vi "SR400_setting.vi"(4 "Counter B Input":enum16{"10 MHz", "INPUT 1", "INPUT 2", "TRIG"}(ring)=enum."INPUT 1", 5 "Counter A Input":enum16{"10 MHz", "INPUT 1", "INPUT 2", "TRIG"}(ring)=enum."INPUT 1", 6 "Gate B delay":dbl[unit], 7 "Number of samples":dbl, 8 "Gate B width":dbl[unit], 9 "Gate A delay":dbl[unit], 10 "Gate A width":dbl[unit], 11 "VISA_SR400":refnum<visa-resource-name>="GPIB0::18::INSTR") -> ()   [LabVIEW 2015]
uses:
  Libraries/SR400/Public/Typedefs/Counter.ctl
  Libraries/SR400/Public/Typedefs/Counting Input.ctl
  Libraries/SR400/Public/Typedefs/Output Source.ctl
  Libraries/SR400/Public/Typedefs/Counter Mode.ctl
  Libraries/SR400/Public/Typedefs/Gate.ctl
  Libraries/SR400/Public/Typedefs/Gate Mode.ctl
  Libraries/SR400/Public/Typedefs/Counter Preset.ctl
  Libraries/SR400/SR400.lvlib
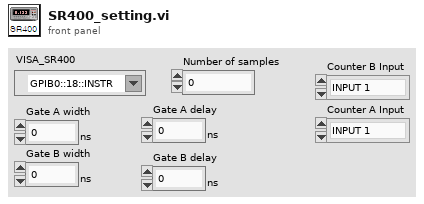
[diagram p1: front panel]
types:
  T1 = typedef "SR400.lvlib/Counter.ctl" = enum16{"Counter A", "Counter B", "Counter T"}
  T2 = typedef "SR400.lvlib/Counter Preset.ctl" = enum16{"Invalid", "Counter B", "Counter T"}
  T3 = typedef "SR400.lvlib/Gate Mode.ctl" = enum16{"CW", "Fixed", "Scan"}
  T4 = typedef "SR400.lvlib/Gate.ctl" = enum16{"Gate A", "Gate B"}
  T5 = typedef "SR400.lvlib/Counter Mode.ctl" = enum16{"A,B For T Preset", "A-B For T Preset", "A+B For T Preset", "A For B Preset"}
  T6 = typedef "SR400.lvlib/Output Source.ctl" = enum16{"A", "B", "A - B", "A + B"}
  T7 = typedef "SR400.lvlib/Counting Input.ctl" = enum16{"10 MHz", "INPUT 1", "INPUT 2", "TRIG"}
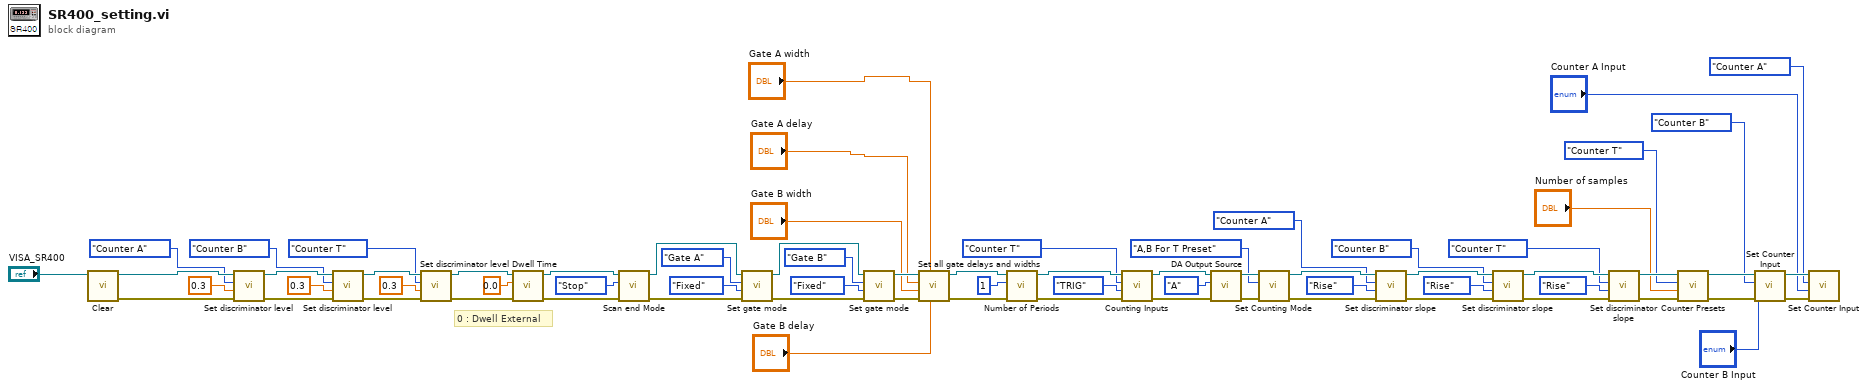
[diagram p0: block diagram]
diagram:
  # "0 : Dwell External"
  n1 = call "Clear.vi"("VISA resource name"="VISA_SR400") -> ("error out"=w33:errorcluster, "VISA resource name out"=w70:refnum<visa-resource-name>)  [unwired: 9 in]
  n2 = call "Set discriminator level.vi"("error in (no error)"=w33, "Level (-0.034 V)"=0.3, "Discriminator (def: A)"=Counter."Counter A", "VISA resource name"=w70) -> ("error out"=w32:errorcluster, "VISA resource name out"=w67:refnum<visa-resource-name>)  [unwired: 6 in]
  n3 = call "Set discriminator level.vi"("error in (no error)"=w32, "Level (-0.034 V)"=0.3, "Discriminator (def: A)"=Counter."Counter B", "VISA resource name"=w67) -> ("error out"=w31:errorcluster, "VISA resource name out"=w64:refnum<visa-resource-name>)  [unwired: 6 in]
  n4 = call "Set discriminator level.vi"("error in (no error)"=w31, "Level (-0.034 V)"=0.3, "Discriminator (def: A)"=Counter."Counter T", "VISA resource name"=w64) -> ("error out"=w18:errorcluster, "VISA resource name out"=w19:refnum<visa-resource-name>)  [unwired: 6 in]
  n5 = call "Dwell Time.vi"("error in (no error)"=w18, "Dwell time (0.002 s)"=0.0, "VISA resource name"=w19) -> ("error out"=w30:errorcluster, "VISA resource name out"=w60:refnum<visa-resource-name>)  [unwired: 7 in]
  n6 = call "Scan end Mode.vi"("error in (no error)"=w30, "Scan End Mode (Def: Stop)"=enum16{"Stop", "Start"}."Stop", "VISA resource name"=w60) -> ("error out"=w29:errorcluster, "VISA resource name out"=w49:refnum<visa-resource-name>)  [unwired: 7 in]
  n7 = call "Set gate mode.vi"("error in (no error)"=w29, "Mode (def: CW)"=Gate_Mode."Fixed", "Gate (def: A)"=Gate."Gate A", "VISA resource name"=w49) -> ("error out"=w28:errorcluster, "VISA resource name out"=w46:refnum<visa-resource-name>)  [unwired: 6 in]
  n8 = call "Set gate mode.vi"("error in (no error)"=w28, "Mode (def: CW)"=Gate_Mode."Fixed", "Gate (def: A)"=Gate."Gate B", "VISA resource name"=w46) -> ("error out"=w27:errorcluster, "VISA resource name out"=w45:refnum<visa-resource-name>)  [unwired: 6 in]
  n9 = call "Set all gate delays and widths.vi"("Gate B Delay (def: 0 s)"="Gate B delay", "Gate A Width (def: 0 s)"="Gate A width", "error in (no error)"=w27, "Gate B Width (def: 0 s)"="Gate B width", "Gate A Delay (def: 0 s)"="Gate A delay", "VISA resource name"=w45) -> ("error out"=w26:errorcluster, "VISA resource name out"=w58:refnum<visa-resource-name>)  [unwired: 4 in]
  n10 = call "Number of Periods.vi"("error in (no error)"=w26, "# of periods (def: 1)"=1, "VISA resource name"=w58) -> ("error out"=w25:errorcluster, "VISA resource name out"=w56:refnum<visa-resource-name>)  [unwired: 7 in]
  n11 = call "Counting Inputs.vi"("error in (no error)"=w25, "j (0)"=Counting_Input."TRIG", "i (0)"=Counter."Counter T", "VISA resource name"=w56) -> ("error out"=w24:errorcluster, "VISA resource name out"=w53:refnum<visa-resource-name>)  [unwired: 6 in]
  n12 = call "DA Output Source.vi"("error in (no error)"=w24, "j (0)"=Output_Source."A", "VISA resource name"=w53) -> ("error out"=w23:errorcluster, "VISA resource name out"=w51:refnum<visa-resource-name>)  [unwired: 7 in]
  n13 = call "Set Counting Mode.vi"("error in (no error)"=w23, "Mode (def: A,B for T preset)"=Counter_Mode."A,B For T Preset", "VISA resource name"=w51) -> ("error out"=w22:errorcluster, "VISA resource name out"=w42:refnum<visa-resource-name>)  [unwired: 7 in]
  n14 = call "Set discriminator slope.vi"("error in (no error)"=w22, "j (0)"=enum16{"Rise", "Fall"}."Rise", "i (0)"=Counter."Counter A", "VISA resource name"=w42) -> ("error out"=w21:errorcluster, "VISA resource name out"=w41:refnum<visa-resource-name>)  [unwired: 6 in]
  n15 = call "Set discriminator slope.vi"("error in (no error)"=w21, "j (0)"=enum16{"Rise", "Fall"}."Rise", "i (0)"=Counter."Counter B", "VISA resource name"=w41) -> ("error out"=w20:errorcluster, "VISA resource name out"=w40:refnum<visa-resource-name>)  [unwired: 6 in]
  n16 = call "Set discriminator slope.vi"("error in (no error)"=w20, "j (0)"=enum16{"Rise", "Fall"}."Rise", "i (0)"=Counter."Counter T", "VISA resource name"=w40) -> ("error out"=w15:errorcluster, "VISA resource name out"=w17:refnum<visa-resource-name>)  [unwired: 6 in]
  n17 = call "Counter Presets.vi"("error in (no error)"=w15, "Number of triggers"="Number of samples", "Counter (Def: T)"=Counter_Preset."Counter T", "VISA resource name"=w17) -> ("error out"=w13:errorcluster, "VISA resource name out"=w14:refnum<visa-resource-name>)  [unwired: 6 in]
  n18 = call "Set Counter Input.vi"("error in (no error)"=w13, "Input (def: 10 MHz)"="Counter B Input", "Counter (def: A)"=Counter."Counter B", "VISA resource name"=w14) -> ("error out"=w10:errorcluster, "VISA resource name out"=w11:refnum<visa-resource-name>)  [unwired: 6 in]
  n19 = call "Set Counter Input.vi"("error in (no error)"=w10, "Input (def: 10 MHz)"="Counter A Input", "Counter (def: A)"=Counter."Counter A", "VISA resource name"=w11) -> ()  [unwired: 6 in, 2 out]
